vi "Return_Current_Coordinates.vi"(6 "error in":errorcluster, 8 "Machine In":refnum<visa-resource-name>, 9 "INPUT Z Coord":dbl, 10 "INPUT X Coord":dbl, 11 "INPUT Y Coord":dbl) -> (0 "x = y?":bool, 1 "OUTPUT Z Coord":dbl, 2 "OUTPUT X Coord":dbl, 3 "OUTPUT Y Coord":dbl, 4 "error out":errorcluster, 5 "Machine Out":refnum<visa-resource-name>)   [LabVIEW 2018]
panel:
  in  "Write Buffer":string
  out "read buffer":string="$22 ok VSwiftPro\r\n$22 ok VSwiftPro\r\n@5 V1\r\n$22 ok VSwiftPro\r\n$22 ok VSwiftPro\r\n$22 ok VSwiftPro\r\n$22 ok VSwiftPro\r\n$22 ok VSwiftPro\r\n$22 ok VSwiftPro\r\n$62 ok X157.66 Y1.93 Z-2.12\r\n$22 ok VSwiftPro\r\nstart\necho:Marlin 1.1.0-RC7\necho: Last Updatstart\necho:Marlin 1.1.0-RC7\necho: Last Updated: 2016-07-31 12:00 | Author: (none, default config)\nCompiled: Oct 25 2017\necho: Free Memory: 2376  PlannerBufferBytes: 924\necho:Hardcoded Default Settings Loaded\necho:Steps per unit:\necho:  M92 X320.00 Y320.00 Z320.00 E84.88\necho:Maximum feedrates (mm/s):\necho:  M203 X2000.00 Y2000.00 Z2000.00 E25.00\necho:Maximum Acceleration (mm/s2):\necho:  M201 X2000 Y2000 Z2000 E10000\necho:Accelerations: P=printing, R=retract and T=travel\necho:  M204 P25.00 R25.00 T100.00\necho:Advanced variables: S=Min feedrate (mm/s), T=Min travel feedrate (mm/s), B=minimum segment time (ms), X=maximum XY jerk (mm/s),  Z=maximum Z jerk (mm/s),  E=maximum E jerk (mm/s)\necho:  M205 S0.00 T0.00 B20000 X1.00 Z1.00 E5.00\necho:Home offset (mm)\necho:  M206 X0.00 Y0.00 Z0.00\necho:PID settings:\necho:  M301 P22.20 I1.08 D114.00\necho:Filament settings: Disabled\necho:  M200 D1.75\necho:  M200 D0\n"
  in  "G Code Command":string="#n P2220\n "
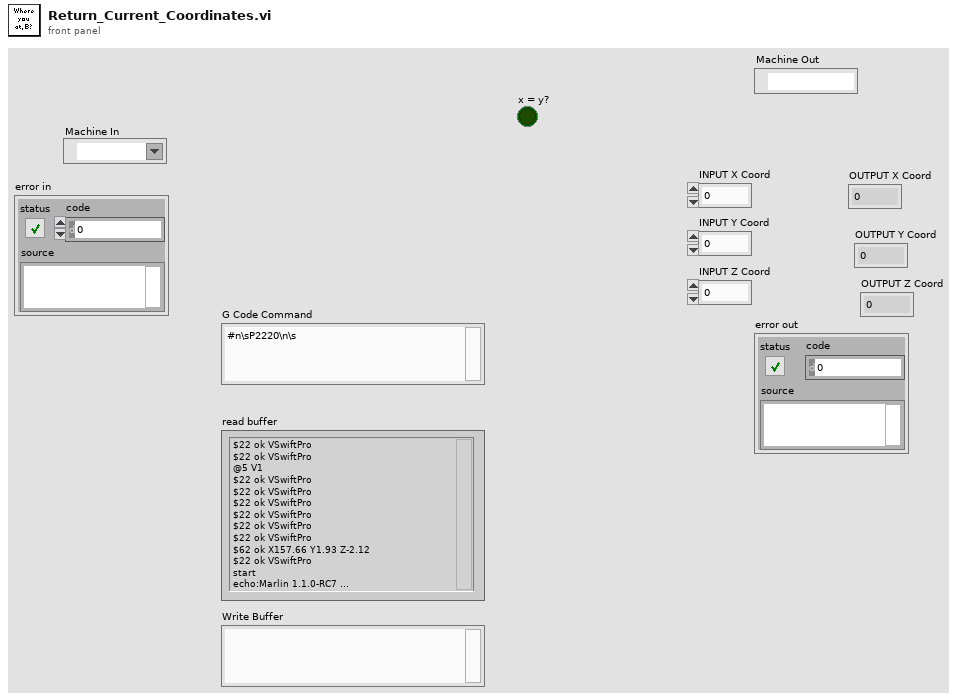
[diagram p1: front panel]
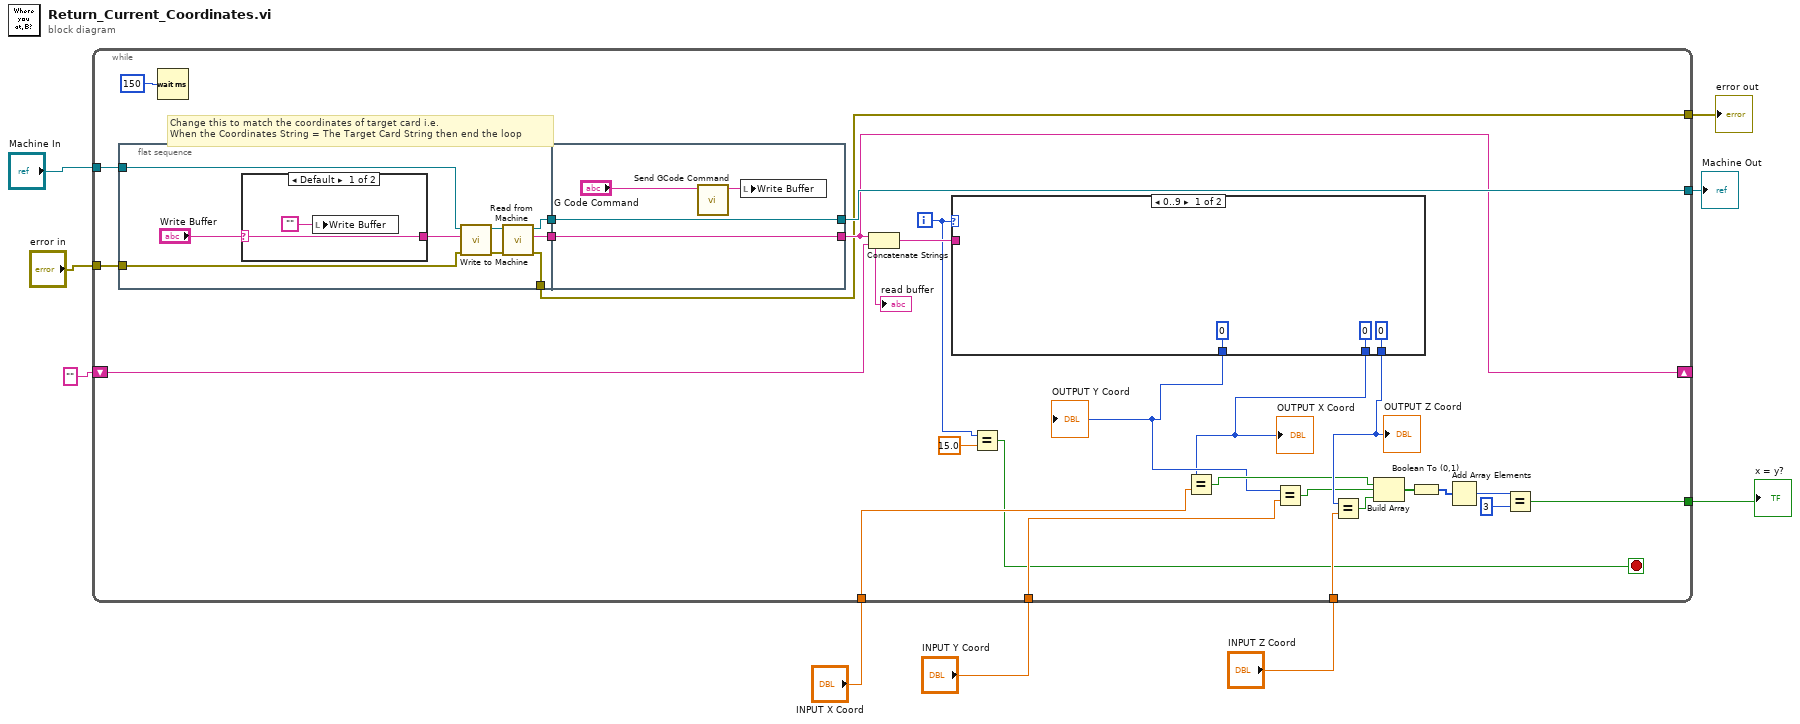
[diagram p0: block diagram]
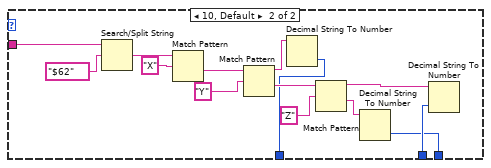
[diagram p2: hidden frame]
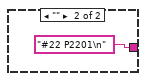
[diagram p3: hidden frame]
diagram:
  n1 = while {
    tunnel: "Machine In" -> [w35]
    tunnel: "error in" -> [w33]
    shift-right: [w29] -> _
    shift-left: "" -> [w34]
    tunnel: [w32] -> w3
    tunnel: "INPUT X Coord" -> [w27]
    tunnel: "INPUT Y Coord" -> [w26]
    tunnel: "INPUT Z Coord" -> [w24]
    tunnel: [w14] -> w2
    tunnel: [w10] -> w1
    i -> [w12]
    stop <- w11 stop-if-true
    # "Change this to match the coordinates of target card i.e.\nWhen the Coordinates String = The Target Card String then end the loop"
    n2 = flat-sequence {
      tunnel: w35 -> [w58]
      tunnel: w33 -> [w56]
      tunnel: [w57] -> w31
      tunnel: [w55] -> w30
      tunnel: [w54] -> w14
      tunnel: [w68] -> w32
      tunnel: [w69] -> w29
      tunnel: w31 -> [w69]
      tunnel: w30 -> [w68]
      frame #0 {
        n3 = case shown="Default" "Write Buffer" {
          selector: "Write Buffer" -> [w64 _]
          tunnel: [w64 "#22 P2201\n"] -> w61
          frame Default {
            n4 = local write "Write Buffer"("") -> ()
          }
          frame "" {
          }
        }
        n5 = call "Write to Machine .vi"("error in (no error)"=w56, "G-Code String In"=w61, "Machine In"=w58) -> ("error out"=w59:errorcluster, "Machine Out"=w60:refnum<visa-resource-name>)  [unwired: 7 in]
        n6 = call "Read from Machine.vi"("error in (no error)"=w59, "Machine In"=w60) -> ("error out"=w54:errorcluster, "read buffer"=w57:string, "Machine Out"=w55:refnum<visa-resource-name>)  [unwired: 7 in]
      }
      frame #1 {
        n7 = call "Send GCode Command.vi"("G-Code Command in"="G Code Command") -> ("G-Code Command out"=w67:string)  [unwired: 10 in]
        n8 = local write "Write Buffer"(w67) -> ()
      }
    }
    n9 = Wait (ms)(milliseconds to wait=u32 150) -> ()  [unwired: 1 out]
    n10 = Concatenate Strings(w29, w34) -> (w28:string)
    "read buffer" <- w28
    n11 = case shown="0..9" w12 {
      tunnel: w28 -> [_ w43]
      tunnel: [0 w42] -> w16
      tunnel: [0 w41] -> w15
      tunnel: [0 w40] -> w25
      frame 0..9 {
      }
      frame 10, Default {
        n12 = Search/Split String(string=w43, search string/char (-)="$62") -> (match + rest of string=w52:string)  [unwired: 1 in, 2 out]
        n13 = Match Pattern(string=w52, regular expression="X") -> (after substring=w48:string)  [unwired: 1 in, 3 out]
        n14 = Match Pattern(string=w48, regular expression="Y") -> (before substring=w47:string, after substring=w46:string)  [unwired: 1 in, 2 out]
        n15 = Decimal String To Number(string=w47) -> (number=w42:i32)  [unwired: 2 in, 1 out]
        n16 = Match Pattern(string=w46, regular expression="Z") -> (before substring=w45:string, after substring=w44:string)  [unwired: 1 in, 2 out]
        n17 = Decimal String To Number(string=w44) -> (number=w40:i32)  [unwired: 2 in, 1 out]
        n18 = Decimal String To Number(string=w45) -> (number=w41:i32)  [unwired: 2 in, 1 out]
      }
    }
    "OUTPUT Y Coord" <- w16
    "OUTPUT X Coord" <- w15
    "OUTPUT Z Coord" <- w25
    n19 = Equal?(x=w12, y=15.0) -> (x = y?=w11:bool)
    n20 = Equal?(x=w15, y=w27) -> (x = y?=w23:bool)
    n21 = Equal?(x=w16, y=w26) -> (x = y?=w22:bool)
    n22 = Equal?(x=w25, y=w24) -> (x = y?=w21:bool)
    n23 = Build Array(w23, w22, w21) -> (w20:bool[])
    n24 = Boolean To (0,1)(Boolean=w20) -> (0, 1=w19:i16[])
    n25 = Add Array Elements(numeric array=w19) -> (sum=w18:i16)
    n26 = Equal?(x=w18, y=i16 3) -> (x = y?=w10:bool)
  }
  "Machine Out" <- w3
  "error out" <- w2
  "x = y?" <- w1
